vi "Add Tests.vi"(8 "error in (no error)":errorcluster, 10 "Tests":string[](array[string]), 11 "Result Model In":refnum<class "Result Model.lvclass">) -> (0 "error out":errorcluster, 3 "Result Model Out":refnum<class "Result Model.lvclass">)   [LabVIEW 2020, in "Result Model.lvclass"]
uses:
  Result Model.lvclass
  Result Model.lvclass/Result Model.ctl
  Core/Result/Status.ctl
  Core/Result/Result.lvlib
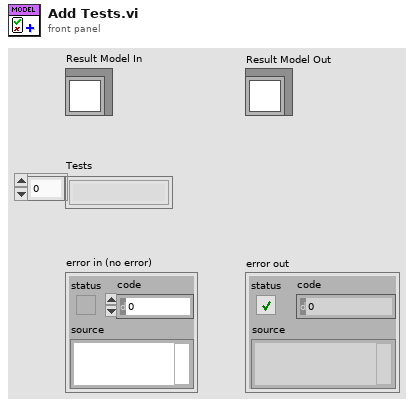
[diagram p1: front panel]
types:
  T1 = typedef "Result.lvlib/Status.ctl" = enum16{"", "Passed", "Failed", "Error", "Skipped", "Setup Error", "Broken", "Teardown Error"}
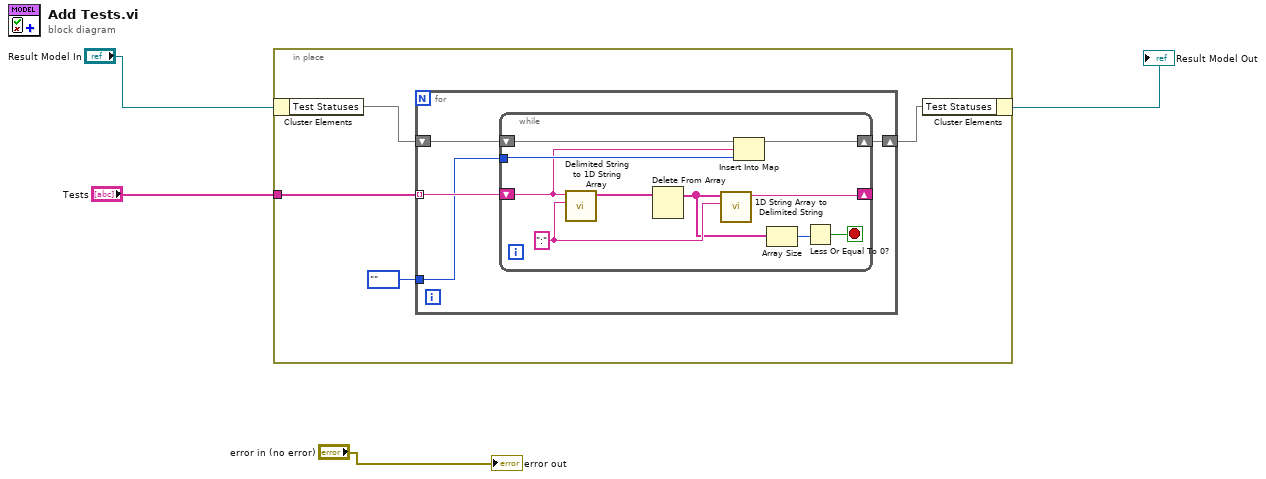
[diagram p0: block diagram]
diagram:
  n1 = in-place {
    in-place-border: "Tests" -> [w8]
    n2 = in-place-cluster #1("Result Model In") -> ("Test Statuses"=w6:map{string, T1})
    n3 = for {
      tunnel: w8 -> [w10] mode=indexing
      shift-right: [w11] -> w5
      shift-left: w6 -> [w12]
      tunnel: Status."" ("Status") -> [w9]
      n4 = while {
        tunnel: w9 -> [w20]
        shift-right: [w21] -> w11
        shift-left: w12 -> [w22]
        shift-right: [w15] -> _
        shift-left: w10 -> [w18]
        stop <- w13 stop-if-true
        w17 = ":" ("delimiter")
        n5 = call <vilib>:"Delimited String to 1D String Array.vi"("delimiter"=w17, "delimited string"=w18) -> ("string array"=w19:string[])  [unwired: 9 in]
        n6 = Delete From Array(array=w19) -> (array with subset deleted=w16:string[])  [unwired: 2 in, 1 out]
        n7 = call <vilib>:"1D String Array to Delimited String.vi"("delimiter"=w17, "string array"=w16) -> ("delimited string"=w15:string)  [unwired: 9 in]
        n8 = Insert Into Map(map in=w22, key=w18, value=w20) -> (map out=w21:map{string, T1})  [unwired: 2 out]
        n9 = Array Size(array=w16) -> (size(s)=w14:i32)
        n10 = Less Or Equal To 0?(x=w14) -> (x <= 0?=w13:bool)
      }
    }
    n11 = in-place-cluster #1("Test Statuses"=w5) -> (→"Result Model Out":refnum<class "Result Model.lvclass">)
  }
  "error out" <- "error in (no error)"
